vi "Write Object Coordinates.vi"(8 "error in (no error)":errorcluster, 10 "Object Coordinates":T1, 11 "Pane Object Position in":refnum<class "Pane Object Position.lvclass">) -> (0 "error out":errorcluster, 3 "Pane Object Position out":refnum<class "Pane Object Position.lvclass">)   [LabVIEW 2018, in "Pane Object Position.lvclass"]
uses:
  Pane Object Position.lvclass
  Object Coordinates.ctl
  Pane Object Position.lvclass/Pane Object Position.ctl
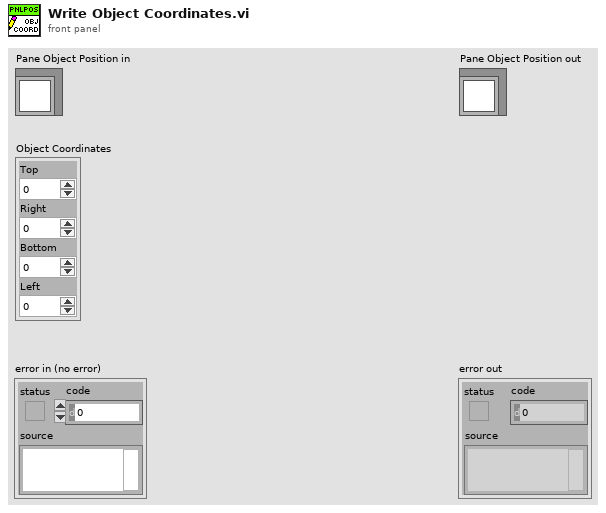
[diagram p1: front panel]
types:
  T1 = typedef "Pane Object Position.lvclass/Object Coordinates.ctl" = cluster{"Top":i32, "Right":i32, "Bottom":i32, "Left":i32}
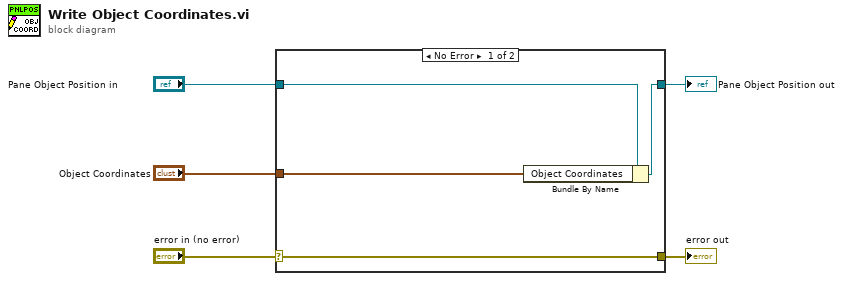
[diagram p0: block diagram]
diagram:
  n1 = case shown="No Error" "error in (no error)" {
    selector: "error in (no error)" -> [w9 w10]
    tunnel: [w9 w10] -> w4
    tunnel: [w7 w11] -> w2
    tunnel: "Pane Object Position in" -> [w8 w11]
    tunnel: "Object Coordinates" -> [w6 _]
    frame No Error {
      n2 = Bundle By Name(cluster=w8, "Object Coordinates"=w6) -> (w7:refnum<class "Pane Object Position.lvclass">)
    }
    frame Error {
    }
  }
  "error out" <- w4
  "Pane Object Position out" <- w2
